vi "Read Child Nodes.vi"(8 "error in (no error)":errorcluster, 11 "Messenger Map Composite in":refnum<class "Messenger Map Composite.lvclass">) -> (0 "error out":errorcluster, 2 "Child Nodes":map{i64, refnum<class "Messenger.lvclass">}(c390), 3 "Messenger Map Composite out":refnum<class "Messenger Map Composite.lvclass">)   [LabVIEW 2024, in "Messenger Map Composite.lvclass"]
uses:
  Messenger Map Composite.lvclass
  Messenger/Messenger.lvclass
  Messenger Map Composite.lvclass/Messenger Map Composite.ctl
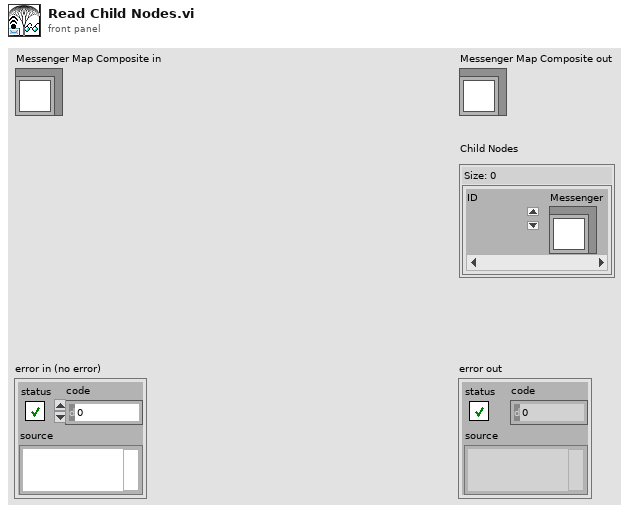
[diagram p1: front panel]
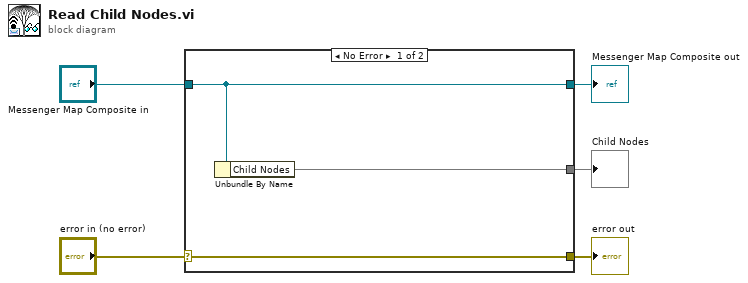
[diagram p0: block diagram]
diagram:
  n1 = case shown="No Error" "error in (no error)" {
    selector: "error in (no error)" -> [w8 w9]
    tunnel: [w8 w9] -> w4
    tunnel: [w7 w10] -> w2
    tunnel: "Messenger Map Composite in" -> [w7 w10]
    tunnel: [w6 _] -> w1
    frame No Error {
      n2 = Unbundle By Name(w7) -> ("Child Nodes"=w6:map{i64, refnum<class "Messenger.lvclass">})
    }
    frame Error {
    }
  }
  "error out" <- w4
  "Messenger Map Composite out" <- w2
  "Child Nodes" <- w1
